vi "React.vi"(8 "error in":errorcluster, 10 "CANopen Message":refnum<class "CANopen Response Message.lvclass">, 11 "CANopen Master in":refnum<class "CANopen Master.lvclass">) -> (0 "error out":errorcluster, 3 "CANopen Master out":refnum<class "CANopen Master.lvclass">)   [LabVIEW 2024, in "CANopen Master.lvlib" / "CANopen Master.lvclass"]
uses:
  CANopen Master.lvclass
  CANopen Master.lvclass/CANopen Master.ctl
  SDO Manager/SDO Manager.lvclass
  CANopen Response/CANopen Response Message.lvclass
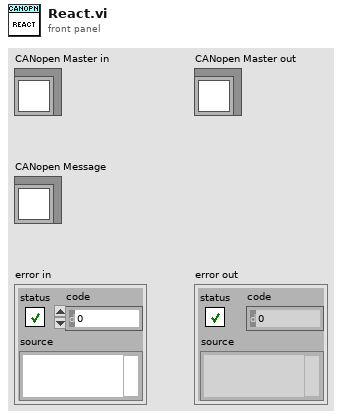
[diagram p1: front panel]
types:
  T1 = typedef "CANopen Master.lvlib/CANopen Response Message.lvclass/Server Command Specifier.ctl" = enum8{"Upload Segment Response", "Download Segment Response", "Initiate Upload Response", "Initiate Download Response", "Heartbeat", "Block Download"}
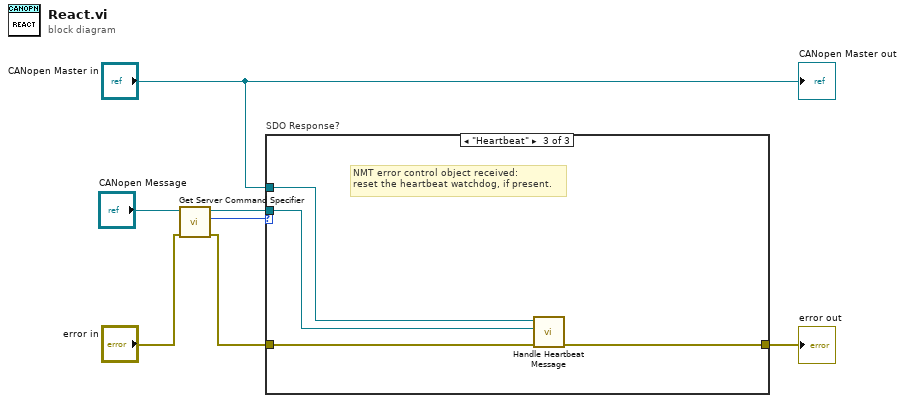
[diagram p0: block diagram]
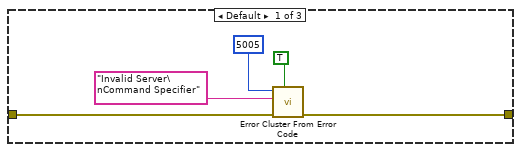
[diagram p2: hidden frame]
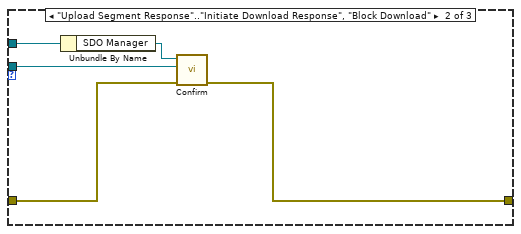
[diagram p3: hidden frame]
diagram:
  n1 = call-dynamic "Get Server Command Specifier.vi"("error in"="error in", "CANopen Response in"="CANopen Message") -> ("error out"=w2:errorcluster, "Server Command Specifier"=w3:T1, "CANopen Response out"=w1:refnum<class "CANopen Response Message.lvclass">)  [unwired: 7 in]
  n2 = case "SDO Response?" shown="\"Heartbeat\"" w3 {
    tunnel: w2 -> [w12 w17 w20]
    tunnel: [w11 w16 w19] -> w7
    tunnel: "CANopen Master in" -> [_ w15 w21]
    tunnel: w1 -> [_ w13 w18]
    frame Default {
      n3 = call <vilib>:"Error Cluster From Error Code.vi"("show call chain? (False)"=TRUE, "error in (no error)"=w12, "error message (\"\")"="Invalid Server\nCommand Specifier" ("error message (\"\")"), "error code (0)"=5005) -> ("error out"=w11:errorcluster)  [unwired: 5 in]
    }
    frame "Upload Segment Response".."Initiate Download Response", "Block Download" {
      n4 = Unbundle By Name(w15) -> ("SDO Manager"=w14:refnum<class "SDO Manager.lvclass">)
      n5 = call "Confirm.vi"("error in"=w17, "CANopen Message"=w13, "SDO Manager in"=w14) -> ("error out"=w16:errorcluster)  [unwired: 7 in, 1 out]
    }
    frame "Heartbeat" {
      # "NMT error control object received:\nreset the heartbeat watchdog, if present."
      n6 = call "Handle Heartbeat Message.vi"("error in"=w20, "CANopen Message"=w18, "CANopen Master in"=w21) -> ("error out"=w19:errorcluster)  [unwired: 7 in, 1 out]
    }
  }
  "error out" <- w7
  "CANopen Master out" <- "CANopen Master in"
